vi "Demo.vi"() -> ()   [LabVIEW 2016]
doc: "This VI demonstrates how to setup a measurement with certain signals, samplerates and filter frequencies. It also shows how to use the VIs that are required to execute a continuous measurement."
uses:
  hw_QX_hwDriverRef.ctl
panel:
  out "6":dbl[](array[numeric])
  out "5":dbl[](array[numeric])
  out "4":dbl[](array[numeric])
  out "Array 2":cluster{i32[], i32[]}[](array[cluster])
  out "Array":timestamp[](array[timestamp])
  out "Numeric 2":i32
  in  "Numeric":dbl=10000.0 min=0.0 max=40000.0 step=100.0
  in  "Path":path=path "F:/0. iAmleoCHO/0.09 Projects_ZCJX/2017/3. 6Y11S_ZMS_液流台&热气台数据采集/ZcDAQ/E/LabviewPrj/曹队/ZcDAQprj/Modules/DAQ-Device/Hardware Drivers/QX/HBM LabVIEW Driver/DLLs/HBM LabVIEW Driver.license"
  in  "FilterFrequency":dbl(ring)=200.0 items=["0.01"=0.01, "0.02"=0.02, "0.05"=0.05, "0.1"=0.1, "0.2"=0.2, "0.5"=0.5, "1"=1.0, "2"=2.0, "5"=5.0, "10"=10.0, "20"=20.0, "50"=50.0, "100"=100.0, "200"=200.0, "500"=500.0, "1000"=1000.0, "2000"=2000.0, "5000"=5000.0, "10000"=10000.0, "20000"=20000.0]
  out "LicenseIsValid":bool
  out "Diagram":waveform(dbl)[](graph)
  in  "Stop":bool
  in  "Index":i32 min=0 max=3 step=1
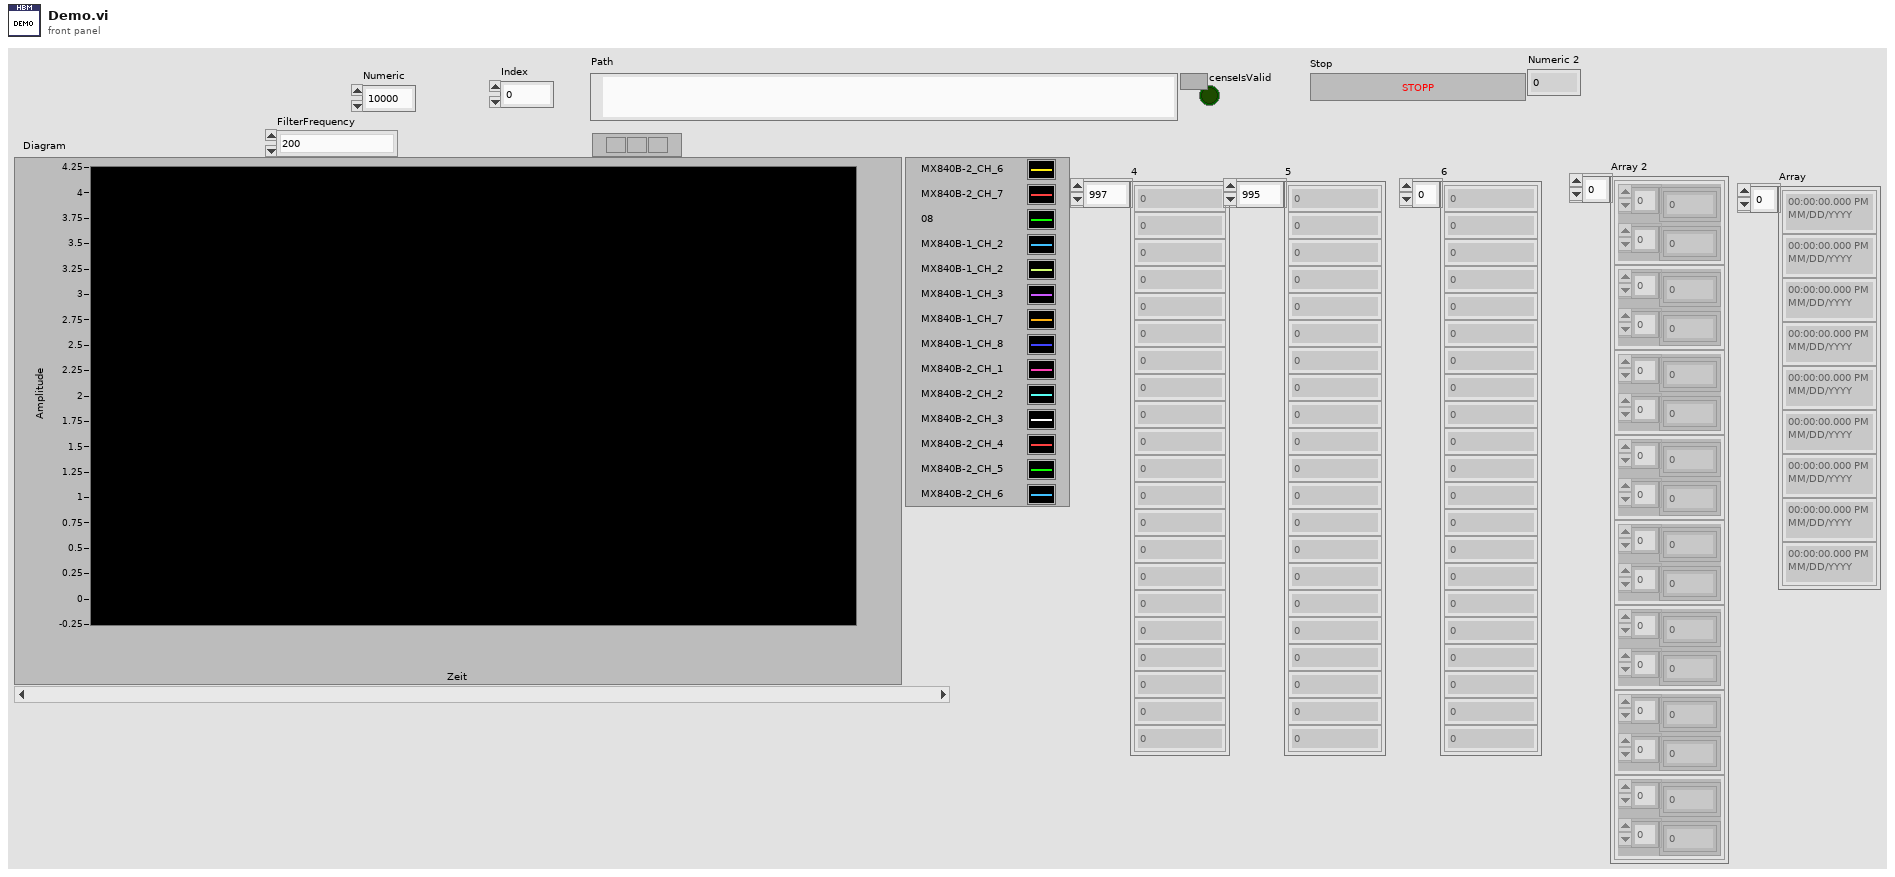
[diagram p1: front panel]
types:
  T1 = typedef "hw_QX_hwDriverRef.ctl" = cluster{"DevicesAndSignals":cluster{"Devices":refnum<k24>[], "Signals":refnum<k24>[]}, "DaqMeasurement":refnum<k24>}
  T2 = enum16{"open", "open or create", "create or replace", "create", "open (read-only)"}
  T3 = cluster{"Devices":refnum<k24>[], "Signals":refnum<k24>[]}
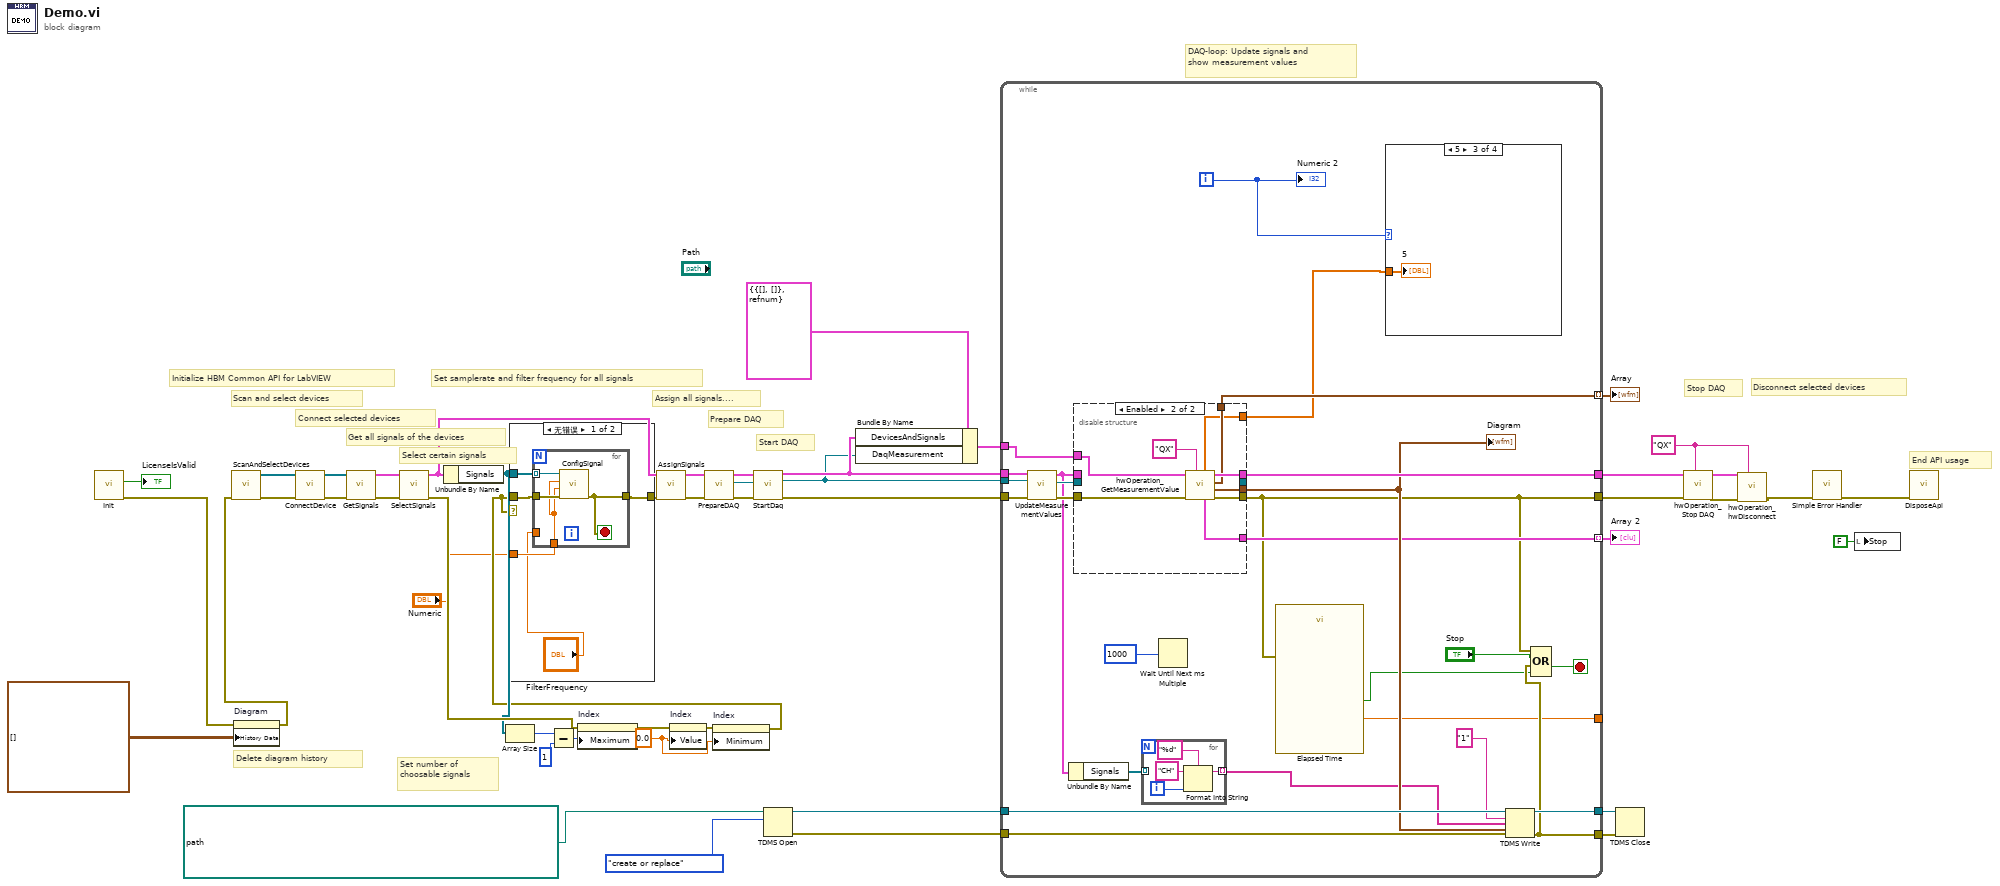
[diagram p0: block diagram]
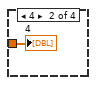
[diagram p4: hidden frame]
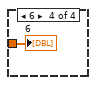
[diagram p5: hidden frame]
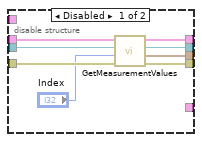
[diagram p6: hidden frame]
diagram:
  w3 = "QX" ("hwType")
  w21 = 0.0 ("Wertebereich:Minimum")
  # "Disconnect selected devices"
  # "Set number of \nchoosable signals"
  # "Delete diagram history"
  # "Initialize HBM Common API for LabVIEW"
  # "End API usage"
  # "Stop DAQ"
  # "DAQ-loop: Update signals and\nshow measurement values"
  # "Start DAQ"
  # "Prepare DAQ"
  # "Select certain signals"
  # "Get all signals of the devices"
  # "Connect selected devices"
  # "Scan and select devices"
  # "Assign all signals...."
  # "Set samplerate and filter frequency for all signals"
  n1 = call "Init.vi"() -> ("LicenseIsValid"=→"LicenseIsValid":bool, "Error out"=w31:errorcluster)  [unwired: 8 in, 1 out]
  n2 = property on="Diagram" class="WFChart (严格)"(error in=w31, "History Data"=waveform(dbl)[][] []) -> (error out=w23:errorcluster)  [unwired: 1 in, 1 out]
  n3 = call "ScanAndSelectDevices.vi"("Error in"=w23) -> ("Error out"=w34:errorcluster, "SelectedDevices"=w35:refnum<k24>[])  [unwired: 8 in, 1 out]
  n4 = call "ConnectDevice.vi"("Error in"=w34, "Devices"=w35) -> ("Error out"=w39:errorcluster, "Devices"=w38:refnum<k24>[])  [unwired: 7 in, 1 out]
  n5 = call "GetSignals.vi"("Error in"=w39, "Devices"=w38) -> ("Error out"=w47:errorcluster, "DevicesAndSignals"=w48:T3)  [unwired: 7 in, 1 out]
  n6 = call "SelectSignals.vi"("error in (no error)"=w47, "DevicesAndSignals"=w48) -> ("error out"=w26:errorcluster, "DevicesAndSignals"=w27:T3)  [unwired: 7 in, 1 out]
  n7 = Unbundle By Name(w27) -> ("Signals"=w24:refnum<k24>[])
  n8 = Array Size(array=w24) -> (size(s)=w30:i32)
  n9 = Subtract(x=w30, y=1) -> (x-y=w28:i32)
  n10 = property on="Index" class="DigNum (严格)"(error in=w26, "Maximum"=w28) -> (error out=w25:errorcluster)  [unwired: 1 in, 1 out]
  n11 = property on="Index" class="DigNum (严格)"(error in=w25, "Value"=w21) -> (error out=w22:errorcluster)  [unwired: 1 in, 1 out]
  n12 = property on="Index" class="DigNum (严格)"(error in=w22, "Minimum"=w21) -> (error out=w20:errorcluster)  [unwired: 1 in, 1 out]
  n13 = case shown="无错误" w20 {
    tunnel: w20 -> [w53 w58]
    tunnel: w24 -> [w52 _]
    tunnel: [w51 w58] -> w46
    tunnel: "Numeric" -> [w50 _]
    frame No Error {
      n14 = for {
        tunnel: w53 -> [w57]
        tunnel: "FilterFrequency" -> [_]
        tunnel: w52 -> [w56] mode=indexing
        tunnel: [w55] -> w51
        tunnel: w50 -> [w54]
        stop <- w55 stop-if-true
        n15 = call "ConfigSignal.vi"("Error in"=w57, "SampleRate"=w54, "FilterFrequency"=w54, "Signal"=w56) -> ("Error out"=w55:errorcluster)  [unwired: 7 in]
      }
    }
    frame Error {
    }
  }
  n16 = call "AssignSignals.vi"("Error in"=w46, "DevicesAndSignals"=w27) -> ("Error out"=w44:errorcluster, "DevicesAndSignals"=w45:T3)  [unwired: 8 in]
  n17 = call "PrepareDAQ.vi"("Error in"=w44, "DevicesAndSignals"=w45) -> ("Error out"=w41:errorcluster, "DaqMeasurement"=w42:refnum<k24>, "DevicesAndSignals"=w43:T3)  [unwired: 7 in]
  n18 = call "StartDaq.vi"("DevicesAndSignals"=w43, "DaqMeasurement"=w42, "Error in"=w41) -> ("DevicesAndSignals"=w10:T3, "DaqMeasurement"=w9:refnum<k24>, "Error out"=w32:errorcluster)  [unwired: 9 in, 1 out]
  n19 = TDMS Open(10:T2."create or replace" ("operation (0:open)"), 11:path "F:/0. iAmleoCHO/0.09 Projects_ZCJX/2017/3. 6Y11S_ZMS_液流台&热气台数据采集/ZcDAQ/E/LabviewPrj/曹队/ZcDAQprj/Builds/TestData/1.tdms" ("file path")) -> (0:w18:errorcluster, 3:w17:refnum<k34>)  [unwired: 5 in]
  n20 = Bundle By Name(cluster=T1 {"DevicesAndSignals"={"Devices"=[], "Signals"=[]}, "DaqMeasurement"=refnum} ("hwDriverRef in"), "DevicesAndSignals"=w10, "DaqMeasurement"=w9) -> (w8:T1)
  n21 = while {
    tunnel: w9 -> [w83]
    tunnel: w10 -> [w82]
    tunnel: [w79] -> w7
    tunnel: w32 -> [w84]
    tunnel: [w61] -> w40
    tunnel: w18 -> [w76]
    tunnel: w17 -> [w77]
    tunnel: [w74] -> w13
    tunnel: [w71] -> w14
    tunnel: w8 -> [w65]
    tunnel: [w64] -> w2 mode=indexing
    tunnel: [w63] -> w1 mode=indexing
    tunnel: [w62] -> _
    i -> [w60]
    stop <- w69 stop-if-true
    n22 = call "UpdateMeasurementValues.vi"("Error in"=w84, "DaqMeasurement"=w83, "DevicesAndSignals"=w82) -> ("Error out"=w80:errorcluster, "DaqMeasurement"=w81:refnum<k24>, "DevicesAndSignals"=w68:T3)  [unwired: 6 in]
    n23 = Unbundle By Name(w68) -> ("Signals"=w67:refnum<k24>[])
    n24 = disable-structure shown="Enabled" {
      disable-tunnel: w68 -> [w99 _]
      disable-tunnel: w81 -> [w98 _]
      disable-tunnel: w80 -> [w97 w108]
      disable-tunnel: [w95 _] -> _
      disable-tunnel: [w94 w105] -> w79
      disable-tunnel: [w93 w106] -> w75
      disable-tunnel: [w92 w107] -> w61
      disable-tunnel: w65 -> [_ w104]
      disable-tunnel: [_ w102] -> w64
      disable-tunnel: [_ w101] -> w63
      disable-tunnel: [_ w100] -> w59
      frame Disabled {
        n25 = call "GetMeasurementValues.vi"("Error in"=w97, "Index"="Index", "DaqMeasurement"=w98, "DevicesAndSignals"=w99) -> ("Error out"=w92:errorcluster, "Waveform"=w93:waveform(dbl), "DaqMeasurement"=w95:refnum<k24>, "DevicesAndSignals"=w94:T3)  [unwired: 4 in]
      }
      frame Enabled {
        n26 = call "hwOperation_GetMeasurementValue.vi"("hwType"="QX", "Error in"=w108, "hwDriverRef in"=w104) -> ("Error out"=w107:errorcluster, "Waveform[]"=w106:waveform(dbl)[], "Time Stamp"=w102:timestamp, "hwDriverRef out"=w105:T1, "Cluster"=w101:cluster{i32[], i32[]}, "Values"=w100:dbl[])  [unwired: 3 in]
      }
    }
    "Diagram" <- w75
    n27 = for {
      tunnel: w67 -> [_] mode=indexing
      tunnel: [w88] -> w66 mode=indexing
      i -> [w91]
      n28 = Format Into String(format string="%d", initial string="CH", w91) -> (resulting string=w88:string)  [unwired: 1 in, 1 out]
    }
    n29 = Wait Until Next ms Multiple(millisecond multiple=u32 1000 ("Vielfache von ms")) -> ()  [unwired: 1 out]
    n30 = call "Elapsed Time"("error in (no error)"=w61) -> ("Elapsed Time (s)"=w62:dbl, "Time has Elapsed"=w70:bool)  [unwired: 11 in, 6 out]
    n31 = case shown="5" w60 {
      tunnel: w59 -> [_ w85 w86 w87]
      frame ..3, Default {
      }
      frame 4 {
        "4" <- w85
      }
      frame 5 {
        "5" <- w86
      }
      frame 6 {
        "6" <- w87
      }
    }
    n32 = TDMS Write(0:w77, 5:"1" ("group name in (Untitled)"), 7:w66, 9:w75, 11:w76) -> (4:w74:refnum<k34>, 15:w71:errorcluster)  [unwired: 1 in, 2 out]
    n33 = Compound Arithmetic op=OR(w61, "Stop", w71, w70) -> (w69:bool)
    "Numeric 2" <- w60
  }
  "Array" <- w2
  "Array 2" <- w1
  n34 = TDMS Close(8:w14, 11:w13) -> ()  [unwired: 2 out]
  n35 = call "hwOperation_Stop DAQ.vi"("hwType"=w3, "error in"=w40, "hwDriverRef in"=w7) -> ("error out"=w6:errorcluster, "hwDriverRef out"=w5:T1)  [unwired: 7 in]
  n36 = call "hwOperation_hwDisconnect.vi"("hwType"=w3, "error in"=w6, "hwDriverRef in"=w5) -> ("error out"=w4:errorcluster)  [unwired: 7 in, 1 out]
  n37 = call <vilib>:"Simple Error Handler.vi"("error in (no error)"=w4) -> ("error out"=w36:errorcluster)  [unwired: 4 in, 4 out]
  n38 = local write "Stop"(FALSE ("Stopp")) -> ()
  n39 = call "DisposeApi.vi"("Error in"=w36) -> ()  [unwired: 10 in, 1 out]
